vi "Read Logs.vi"(8 "error in (no error)":errorcluster, 11 "ModuleAbstract in":refnum<class "ModuleAbstract.lvclass">) -> (0 "error out":errorcluster, 2 "Logs":T1, 3 "ModuleAbstract out":refnum<class "ModuleAbstract.lvclass">)   [LabVIEW 2019, in "ModuleAbstract.lvlib" / "ModuleAbstract.lvclass"]
uses:
  ModuleAbstract.lvclass
  SubModules/EventLog/EventLog.lvclass
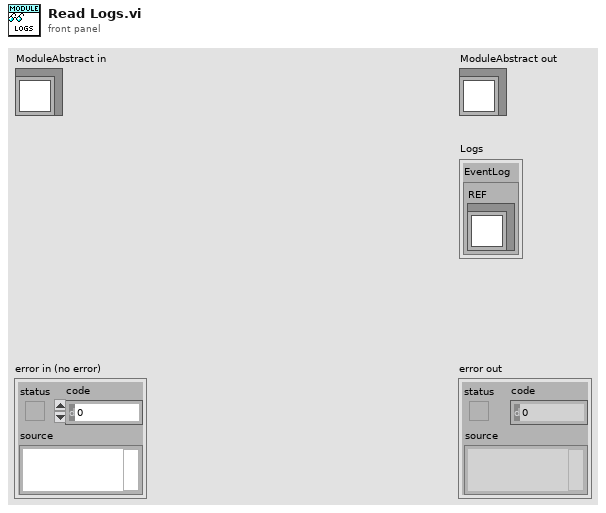
[diagram p1: front panel]
types:
  T1 = cluster{"EventLog":cluster{"REF":refnum<class "EventLog.lvclass">}}
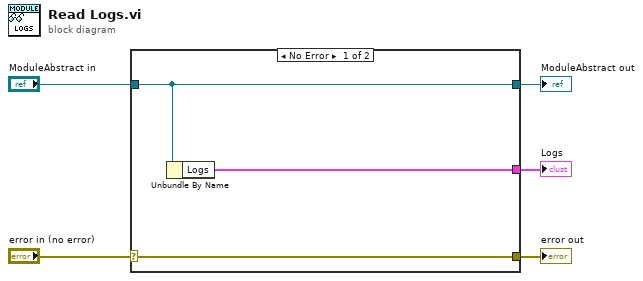
[diagram p0: block diagram]
diagram:
  n1 = case shown="No Error" "error in (no error)" {
    selector: "error in (no error)" -> [w8 w9]
    tunnel: [w8 w9] -> w4
    tunnel: [w7 w10] -> w2
    tunnel: "ModuleAbstract in" -> [w7 w10]
    tunnel: [w6 _] -> w1
    frame No Error {
      n2 = Unbundle By Name(w7) -> ("Logs"=w6:T1)
    }
    frame Error {
    }
  }
  "error out" <- w4
  "ModuleAbstract out" <- w2
  "Logs" <- w1
